vi "stage_calibration_todo demo.vi"() -> ()   [LabVIEW 2024]
uses:
  <vilib>/Utility/file.llb/Read From Spreadsheet File (DBL).vi
panel:
  in  "Unit":bool
  in  "MeasurementRate":dbl=100.0
  in  "Done moving":bool
  out "Manual waiting":bool=TRUE
  in  "Manual":bool=TRUE
  out "Sensor Angle":dbl[](array[numeric])=[116.67480468749802, 1.1645507812499802, -17.29248046874971]
  out "Sensor Position":dbl[](array[numeric])=[86.72958984374999, 336.76083984375, -29.13310546875]
  in  "Acq. Sensor":i32
  in  "Sensor type":enum16{"3D guidance", "ASAP", "ILEMT"}(ring)=enum."ILEMT"
  in  "Settling time":dbl=10.0
  out "Out OK":bool
  out "In OK":bool
  in  "Run":bool
  in  "Input mode":enum16{"Absolute axis", "Relative axis", "Pose"}(ring)=enum."Pose"
  out "Points done":i32
  out "# Points":i32
  out "Position":dbl[](array[numeric]) format="%#_3p"
  out "State":T1(ring)
  in  "Axis names":string[](array[string])=["X", "Y", "Z", "Rx", "Ry", "Rz"]
  in  "Axis enable":bool[](array[boolean])=[TRUE, TRUE, TRUE, TRUE, TRUE, TRUE]
  in  "stop":bool
  in  "Point time":dbl=20.0
  out "ASAP status":cluster{"Valid position":bool, "Message":string}
  in  "Output file":path=path "D:/ilemt_interfere_data/cal_smallerdata_pattern_y0_out.dat"
  in  "Input points file":path=path "D:/ilemt_interfere_data/input_patterns/cal_smallerdata_pattern_y0.dat"
  # "Calibration motion controller"
  # "Point"
  # "of"
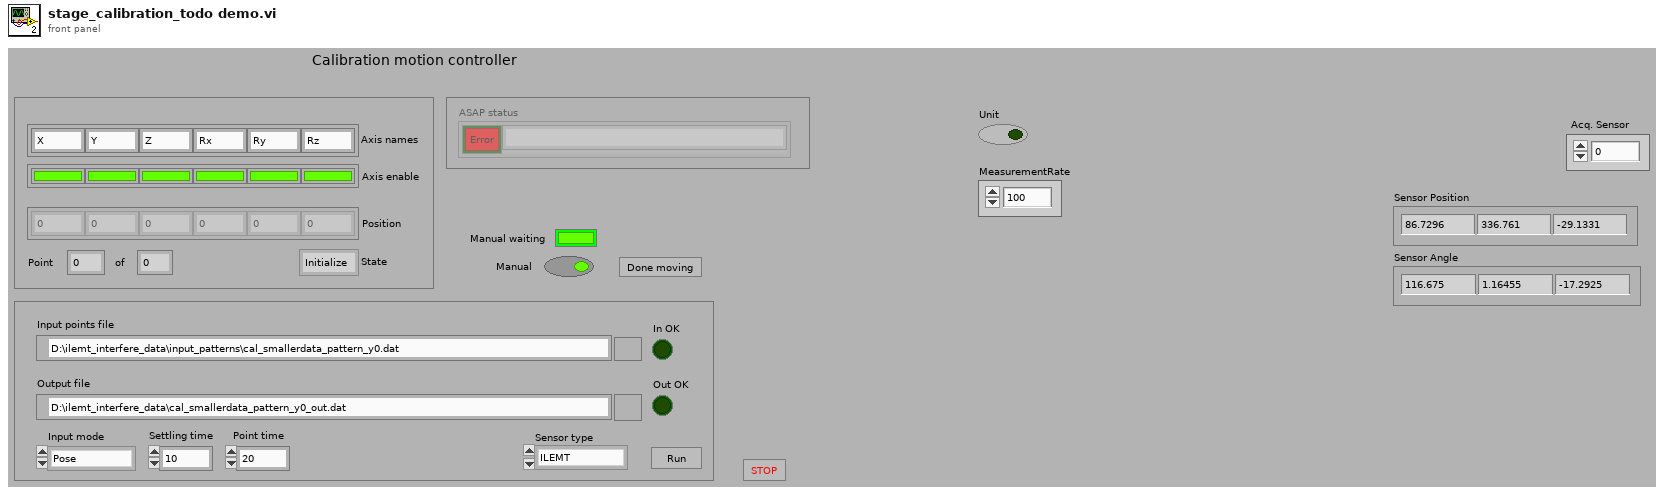
[diagram p1: front panel]
types:
  T1 = enum16{"Initialize", "Move", "Log", "Done", "Error"}
  T2 = enum16{"open", "replace", "create", "open or create", "replace or create", "replace or create with confirmation"}
  T3 = typedef "motion_status.ctl" = cluster{"Axis names":string[], "Axis positions":dbl[], "Pose":dbl[], "Timestamp":u32, "Ready":bool, "Stopped":bool}
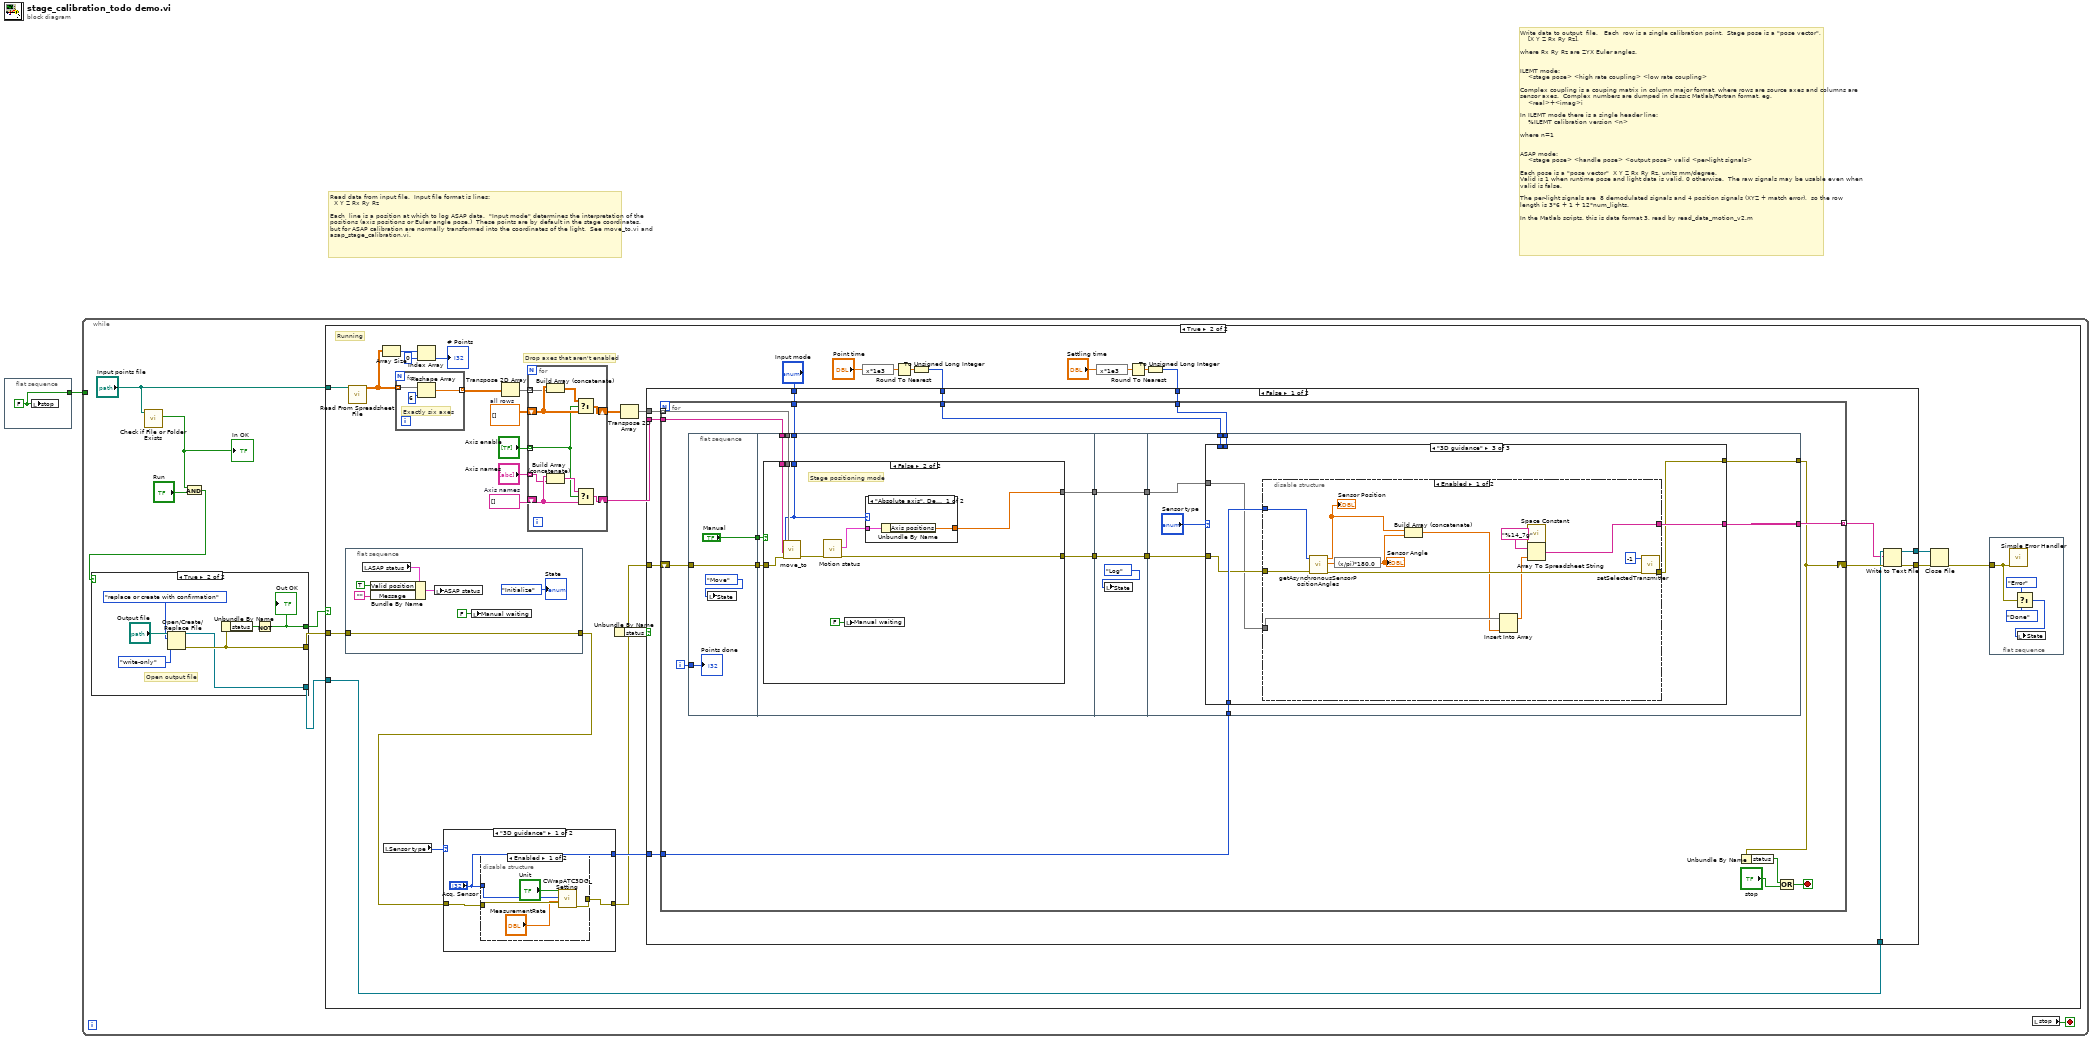
[diagram p0: block diagram]
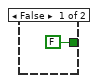
[diagram p2: hidden frame]
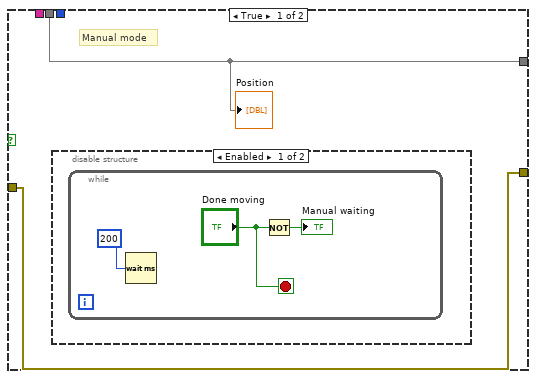
[diagram p6: hidden frame]
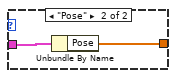
[diagram p8: hidden frame]
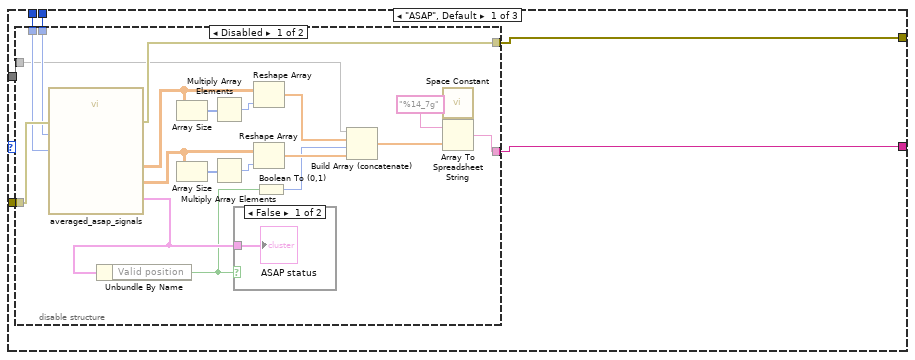
[diagram p9: hidden frame]
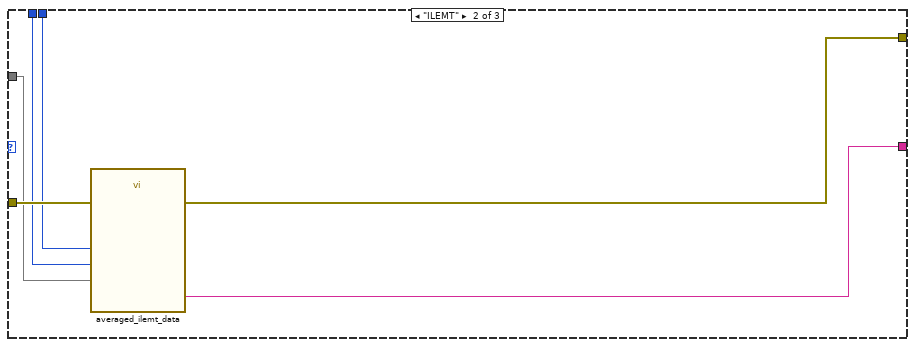
[diagram p12: hidden frame]
diagram:
  # "Write data to output  file.   Each  row is a single calibration point.  Stage pose is a \"pose vector\",\n    [X Y Z Rx Ry Rz],\n\nwhere Rx Ry Rz are ZYX Euler angles.\n\n\nILEMT mode:\n    <stage pose> <high rate coupling> <low rate coupling>\n\nComplex coupling is a couping matrix in column major format, where rows are source axes and columns are sensor axes.  Complex numbers are dumped in classic Matlab/Fortran format, eg. \n    <real>+<imag>i\n\nIn ILEMT mode there is a single header line:\n    %ILEMT calibration version <n>\n\nwhere n=1\n\n\nASAP mode:\n    <stage pose> <handle pose> <output pose> valid <per-light signals>\n\nEach pose is a \"pose vector\"  X Y Z Rx Ry Rz, units mm/degree.\nValid is 1 when runtime pose and light data is valid, 0 otherwise.  The raw signals may be usable even when valid is false.\n\nThe per-light signals are  8 demodulated signals and 4 position signals (XYZ + match error),  so the row length is 3*6 + 1 + 12*num_lights.\n\nIn the Matlab scripts, this is data format 3, read by read_data_motion_v2.m"
  # "Read data from input file.  Input file format is lines:\n  X Y Z Rx Ry Rz\n\nEach  line is a position at which to log ASAP data.  \"Input mode\" determines the interpretation of the positions (axis positions or Euler angle pose.)  These points are by default in the stage coordinates, but for ASAP calibration are normally transformed into the coordinates of the light.  See move_to.vi and asap_stage_calibration.vi."
  n1 = flat-sequence {
    tunnel: [w2] -> w1
    frame #0 {
      w2 = FALSE ("stop")
      n2 = local write "stop"(w2) -> ()
    }
  }
  n3 = while {
    tunnel: w1 -> [_]
    stop <- w7 stop-if-true
    n4 = call <vilib>:"Check if File or Folder Exists.vi"("path"="Input points file") -> ("file or folder exists?"=w3:bool)  [unwired: 8 in, 2 out]
    "In OK" <- w3
    n5 = And(x=w3, y="Run") -> (x .and. y?=w5:bool)
    n6 = case shown="True" w5 {
      tunnel: [_ w18] -> w9
      tunnel: [_ w17] -> w8
      tunnel: [FALSE w12] -> w4
      frame False {
      }
      frame True {
        # "Open output file"
        n7 = Open/Create/Replace File(file path (use dialog)="Output file", operation (0:open)=T2."replace or create with confirmation", access (0:read/write)=enum16{"read/write", "read-only", "write-only"}."write-only") -> (refnum out=w17:refnum<file>, error out=w18:errorcluster)  [unwired: 3 in, 1 out]
        n8 = Unbundle By Name(w18) -> ("status"=w16:bool)
        n9 = Not(x=w16) -> (.not. x?=w12:bool)
        "Out OK" <- w12
      }
    }
    n10 = case shown="True" w4 {
      tunnel: "Input points file" -> [_ w50]
      tunnel: w9 -> [_ w22]
      tunnel: w8 -> [_ w36]
      frame False {
        # "Don't run"
      }
      frame True {
        w43 = string[] []  # Axis names
        w46 = dbl[][] []  # all rows
        # "Running"
        # "Drop axes that aren't enabled"
        n11 = flat-sequence {
          tunnel: w22 -> [w71]
          tunnel: [w71] -> w20
          frame #0 {
            n12 = local read "ASAP status"() -> (w67:cluster{"Valid position":bool, "Message":string})
            n13 = Bundle By Name(cluster=w67, "Valid position"=TRUE, "Message"="") -> (w69:cluster{"Valid position":bool, "Message":string})
            n14 = local write "ASAP status"(w69) -> ()
            n15 = local write "Manual waiting"(FALSE ("Manual waiting")) -> ()
            "State" <- enum16{"Initialize", "Move", "Log", "Done"}."Initialize" ("State")
          }
        }
        n16 = call-poly <vilib>:"Read From Spreadsheet File.vi"("file path (dialog if empty)"=w50) -> ("all rows"=w34:dbl[][])  [unwired: 6 in, 4 out]
        n17 = Array Size(array=w34) -> (size(s)=w39:i32[])
        n18 = local read "Sensor type"() -> (w21:enum16{"3D guidance", "ASAP", "ILEMT"})
        n19 = for {
          tunnel: w34 -> [w64] mode=indexing
          tunnel: [w62] -> w32 mode=indexing
          # "Exactly six axes"
          n20 = Reshape Array "Reshape Array"(w64, 6 ("dimension size")) -> (w62:dbl[])
        }
        n21 = Index Array(array=w39, index=0) -> (element=→"# Points":i32)
        n22 = case shown="\"3D guidance\"" w21 {
          tunnel: [w54 w61] -> w19
          tunnel: ["Acq. Sensor" _] -> w23
          tunnel: w20 -> [w52 w61]
          frame "3D guidance" {
            n23 = disable-structure shown="Enabled" {
              disable-tunnel: [w59 w60] -> w54
              disable-tunnel: "Acq. Sensor" -> [w55 _]
              disable-tunnel: w52 -> [w58 w60]
              frame Enabled {
                n24 = call "CWrapATC3DG_Setting.vi"("error in"=w58, "MeasurementRate"="MeasurementRate", "Acq. Sensor"=w55, "Unit"="Unit") -> ("error out"=w59:errorcluster)  [unwired: 7 in]
              }
              frame Disabled {
              }
            }
          }
          frame "ASAP", Default {
          }
        }
        n25 = Transpose 2D Array(2D array=w32) -> (transposed array=w44:dbl[][])
        n26 = for {
          shift-right: [w81] -> w38
          shift-left: w46 -> [w84]
          tunnel: "Axis enable" -> [w76] mode=indexing
          tunnel: w44 -> [w83] mode=indexing
          shift-right: [w77] -> w41
          shift-left: w43 -> [w79]
          tunnel: "Axis names" -> [w78] mode=indexing
          n27 = Build Array (concatenate) "Build Array"(w84, w83) -> (w82:dbl[][])
          n28 = Build Array (concatenate) "Build Array"(w79, w78) -> (w80:string[])
          n29 = Select(t=w82, s=w76, f=w84) -> (s? t:f=w81:dbl[][])
          n30 = Select(t=w80, s=w76, f=w79) -> (s? t:f=w77:string[])
        }
        n31 = Unbundle By Name(w19) -> ("status"=w51:bool)
        n32 = Transpose 2D Array(2D array=w38) -> (transposed array=w37:dbl[][])
        n33 = expression code="x*1e3"("Point time") -> (w30:dbl)
        n34 = Round To Nearest(number=w30) -> (nearest integer value=w29:dbl)
        n35 = To Unsigned Long Integer(number=w29) -> (unsigned 32bit integer=w28:u32)
        n36 = expression code="x*1e3"("Settling time") -> (w26:dbl)
        n37 = Round To Nearest(number=w26) -> (nearest integer value=w27:dbl)
        n38 = To Unsigned Long Integer(number=w27) -> (unsigned 32bit integer=w24:u32)
        n39 = case shown="False" w51 {
          tunnel: w19 -> [w92 w208]
          tunnel: w36 -> [w91 w209]
          tunnel: w37 -> [w96 _]
          tunnel: [w95 w209] -> w49
          tunnel: [w93 w208] -> w48
          tunnel: w41 -> [w90 _]
          tunnel: "Input mode" -> [w89 _]
          tunnel: w28 -> [w88 _]
          tunnel: w24 -> [w87 _]
          tunnel: w23 -> [w85 _]
          frame False {
            n40 = for {
              tunnel: w96 -> [w107] mode=indexing
              tunnel: [w115] -> w86 mode=indexing
              shift-right: [w106] -> w94
              shift-left: w92 -> [w114]
              tunnel: w90 -> [w109]
              tunnel: w89 -> [w104]
              tunnel: w88 -> [w102]
              tunnel: w87 -> [w101]
              tunnel: w85 -> [w97]
              i -> [w105]
              stop <- w103 stop-if-true
              n41 = flat-sequence {
                tunnel: w114 -> [w119]
                tunnel: [w119] -> w111
                tunnel: w105 -> [w117]
                tunnel: ["Manual"] -> w98
                tunnel: w111 -> [w126]
                tunnel: [w123] -> w110
                tunnel: w109 -> [w125]
                tunnel: w107 -> [w124]
                tunnel: w104 -> [w122]
                tunnel: [w121] -> w100
                tunnel: w98 -> [w120]
                tunnel: w110 -> [w147]
                tunnel: [w147] -> w108
                tunnel: w100 -> [w145]
                tunnel: [w145] -> w99
                tunnel: [w154] -> w115
                tunnel: w108 -> [w153]
                tunnel: [w155] -> w106
                tunnel: w102 -> [w152]
                tunnel: w101 -> [w151]
                tunnel: w99 -> [w150]
                tunnel: w97 -> [w148]
                frame #0 {
                  n42 = local write "State"(enum16{"Initialize", "Move", "Log", "Done"}."Move" ("State")) -> ()
                  "Points done" <- w117
                }
                frame #1 {
                  n43 = case shown="False" w120 {
                    tunnel: w126 -> [w128 w140]
                    tunnel: w125 -> [_ w139]
                    tunnel: w124 -> [w127 w138]
                    tunnel: [w128 w136] -> w123
                    tunnel: w122 -> [_ w135]
                    tunnel: [w127 w133] -> w121
                    frame True {
                      # "Manual mode"
                      n44 = disable-structure shown="Enabled" {
                        frame Enabled {
                          n45 = while {
                            stop <- "Done moving" stop-if-true
                            n46 = Wait (ms)(milliseconds to wait=200) -> ()  [unwired: 1 out]
                            n47 = Not(x="Done moving") -> (.not. x?=→"Manual waiting":bool)
                          }
                        }
                        frame Disabled {
                        }
                      }
                      "Position" <- w127
                    }
                    frame False {
                      # "Stage positioning mode"
                      n48 = call "move_to.vi"("Error in"=w140, "Axis names"=w139, "Axis positions"=w138, "Mode"=w135) -> ("Error out"=w137:errorcluster)  [unwired: 7 in]
                      n49 = call "Motion status.vi"("error in"=w137) -> ("error out"=w136:errorcluster, "Motion status"=w134:T3)  [unwired: 5 in, 4 out]
                      n50 = local write "Manual waiting"(FALSE ("Manual waiting")) -> ()
                      n51 = case shown="\"Absolute axis\", Default" w135 {
                        tunnel: w134 -> [w142 w144]
                        tunnel: [w141 w143] -> w133
                        frame "Absolute axis", Default {
                          n52 = Unbundle By Name(w142) -> ("Axis positions"=w141:dbl[])
                        }
                        frame "Pose" {
                          n53 = Unbundle By Name(w144) -> ("Pose"=w143:dbl[])
                        }
                      }
                    }
                  }
                }
                frame #2 {
                  n54 = local write "State"(enum16{"Initialize", "Move", "Log", "Done"}."Log" ("State")) -> ()
                }
                frame #3 {
                  n55 = case shown="\"3D guidance\"" "Sensor type" {
                    tunnel: [w161 w187 w190] -> w155
                    tunnel: [w156 w186 w192] -> w154
                    tunnel: w153 -> [w160 w188 w191]
                    tunnel: w152 -> [w159 w184 _]
                    tunnel: w151 -> [w158 w185 _]
                    tunnel: w150 -> [w157 w183 w189]
                    tunnel: w148 -> [_ _ w193]
                    frame "ASAP", Default {
                      n56 = disable-structure shown="Disabled" {
                        disable-tunnel: [w181 _] -> w161
                        disable-tunnel: w160 -> [w179 _]
                        disable-tunnel: w159 -> [w174 _]
                        disable-tunnel: w158 -> [w173 _]
                        disable-tunnel: w157 -> [w167 _]
                        disable-tunnel: [w162 _] -> w156
                        frame Disabled {
                          n57 = call "averaged_asap_signals.vi"("error in"=w179, "Averaging time (ms)"=w174, "Settling time (ms)"=w173) -> ("error out"=w181:errorcluster, "ASAP diagnostics"=w180:cluster{"Valid position":bool, "Message":string}, "Poses"=w166:sgl[][], "Demodulated averaged"=w176:sgl[][])  [unwired: 5 in]
                          n58 = Unbundle By Name(w180) -> ("Valid position"=w172:bool)
                          n59 = Array Size(array=w166) -> (size(s)=w169:i32[])
                          n60 = Array Size(array=w176) -> (size(s)=w178:i32[])
                          n61 = Multiply Array Elements(1:w169) -> (0:w170:i32)
                          n62 = Multiply Array Elements(1:w178) -> (0:w177:i32)
                          n63 = case shown="False" w172 {
                            tunnel: w180 -> [w182 _]
                            frame False {
                              "ASAP status" <- w182
                            }
                            frame True {
                            }
                          }
                          n64 = Reshape Array(w166, w170) -> (w168:sgl[])
                          n65 = Reshape Array(w176, w177) -> (w175:sgl[])
                          n66 = Boolean To (0,1)(Boolean=w172) -> (0, 1=w171:i16)
                          n67 = Build Array (concatenate)(w167, w168, w171, w175) -> (w163:dbl[])
                          n68 = call <vilib>:"Space Constant.vi"() -> ("String"=w164:string)
                          n69 = Array To Spreadsheet String(delimiter (Tab)=w164, array=w163, 3:"%14_7g" ("format (%.3f)")) -> (spreadsheet string=w162:string)
                        }
                        frame Enabled {
                        }
                      }
                    }
                    frame "ILEMT" {
                      n70 = call "averaged_ilemt_data.vi"("error in"=w188, "Position"=w183, "Point time (ms)"=w184, "Settling time (ms)"=w185) -> ("error out"=w187:errorcluster, "Result string"=w186:string)  [unwired: 4 in, 2 out]
                    }
                    frame "3D guidance" {
                      n71 = disable-structure shown="Enabled" {
                        disable-tunnel: [w206 _] -> w190
                        disable-tunnel: w193 -> [w195 _]
                        disable-tunnel: w191 -> [w194 _]
                        disable-tunnel: [w200 _] -> w192
                        disable-tunnel: w189 -> [w199 _]
                        frame Enabled {
                          n72 = call "getAsynchronousSensorPositionAngles.vi"("error in"=w194, "sensorNum"=w195) -> ("error out"=w205:errorcluster, "ang"=w204:dbl[], "pos"=w196:dbl[])  [unwired: 7 in]
                          "Sensor Position" <- w196
                          n73 = expression code="(x/pi)*180.0" ("radians to degrees")(w204) -> (w203:dbl[])
                          "Sensor Angle" <- w203
                          n74 = Build Array (concatenate)(w196, w203) -> (w198:dbl[])
                          n75 = Insert Into Array(array=w199, new element=w198) -> (w197:dbl[])  [unwired: 1 in]
                          n76 = call <vilib>:"Space Constant.vi"() -> ("String"=w201:string)
                          n77 = Array To Spreadsheet String(delimiter (Tab)=w201, array=w197, 3:"%14_7g" ("format (%.3f)")) -> (spreadsheet string=w200:string)
                          n78 = call "setSelectedTransmitter.vi"("error in (no error)"=w205, "transmitterNum"=-1) -> ("error out"=w206:errorcluster)  [unwired: 9 in]
                        }
                        frame Disabled {
                        }
                      }
                    }
                  }
                }
              }
              n79 = Unbundle By Name(w106) -> ("status"=w113:bool)
              n80 = Compound Arithmetic op=OR(w113, "stop") -> (w103:bool)
            }
            n81 = Write to Text File(file (use dialog)=w91, text=w86, error in=w94) -> (refnum out=w95:refnum<file>, error out=w93:errorcluster)  [unwired: 1 in, 1 out]
          }
          frame True {
          }
        }
        n82 = Close File(refnum=w49, error in=w48) -> (error out=w47:errorcluster)  [unwired: 1 out]
        n83 = flat-sequence {
          tunnel: w47 -> [w75]
          frame #0 {
            n84 = call <vilib>:"Simple Error Handler.vi"("error in (no error)"=w75) -> ()  [unwired: 4 in, 5 out]
            n85 = Select(t=T1."Error" ("State"), s=w75, f=T1."Done" ("State")) -> (s? t:f=w72:T1)
            n86 = local write "State"(w72) -> ()
          }
        }
      }
    }
    n87 = local read "stop"() -> (w7:bool)
  }
